vi "VNA_OPEN.vi"(8 "error in (no error)":errorcluster, 9 "Clear Error w/ Report?":bool, 10 "Configuration Cluster":T1={"General"={"Config.ini"=path "", "Default Logging Path"=path ""}, "Hardware"={"Global T VAR"="", "Global B VAR"="", "VISAS"={"GEN COM"="", "SCOPE COM"="", "VNA COM"=""}, "Connected?"={"SCOPE"=FALSE, "GEN"=FALSE, "VNA"=FALSE}}, "Operation"={"Operation Mode"=enum."Idle-Off", "Status"="", "NewLog?"=FALSE, "OvenWarn"=FALSE, "Scope Settings"={"TimeBase"=0.0, "VerticalScale"=4.0, "Channel"=enum."Channel 2"}, "Gen Settings"={"Amplitude"=0.0, "Frequency"=0.0, "Offset"=0.0}}}) -> (0 "error out":errorcluster, 1 "Success?":bool, 2 "Configuration Cluster Out":T1={"General"={"Config.ini"=path "", "Default Logging Path"=path ""}, "Hardware"={"Global T VAR"="", "Global B VAR"="", "VISAS"={"GEN COM"="", "SCOPE COM"="", "VNA COM"=""}, "Connected?"={"SCOPE"=FALSE, "GEN"=FALSE, "VNA"=FALSE}}, "Operation"={"Operation Mode"=enum."Idle-Off", "Status"="", "NewLog?"=FALSE, "OvenWarn"=FALSE, "Scope Settings"={"TimeBase"=0.0, "VerticalScale"=4.0, "Channel"=enum."Channel 2"}, "Gen Settings"={"Amplitude"=0.0, "Frequency"=0.0, "Offset"=0.0}}}, 4 "message":string)   [LabVIEW 2021]
uses:
  Config_Cluster.ctl
  Mode_Enum.ctl
  <vilib>/Utility/error.llb/DialogType.ctl
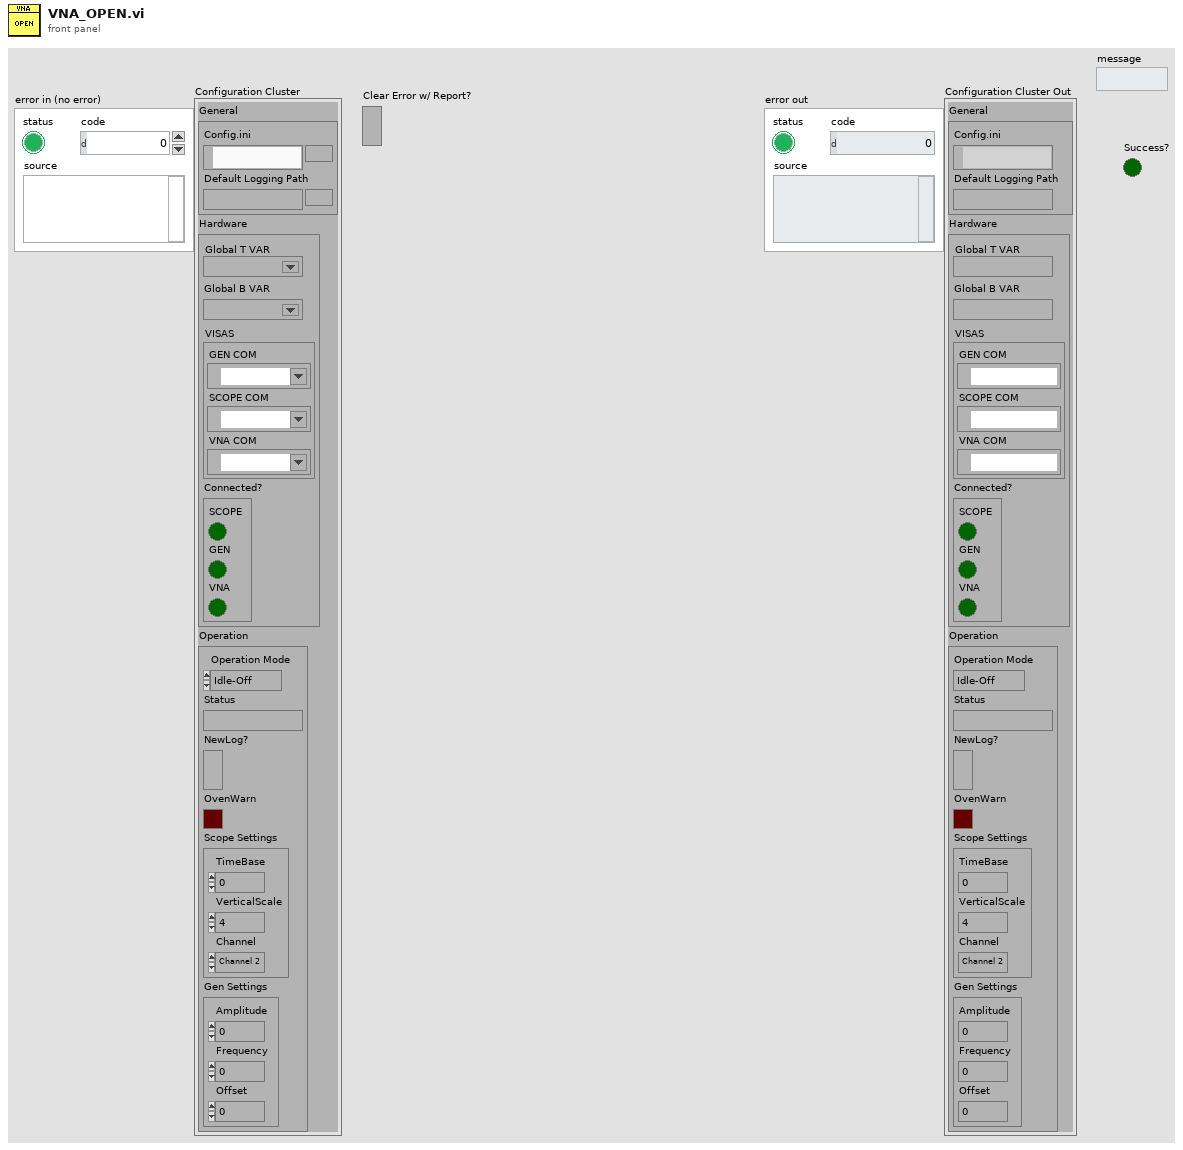
[diagram p1: front panel]
types:
  T1 = typedef "Config_Cluster.ctl" = cluster{"General":cluster{"Config.ini":path, "Default Logging Path":path}, "Hardware":cluster{"Global T VAR":refnum<k21>, "Global B VAR":refnum<k21>, "VISAS":cluster{"GEN COM":refnum<visa-resource-name>, "SCOPE COM":refnum<visa-resource-name>, "VNA COM":refnum<visa-resource-name>}, "Connected?":cluster{"SCOPE":bool, "GEN":bool, "VNA":bool}}, "Operation":cluster{"Operation Mode":T2, "Status":string, "NewLog?":bool, "OvenWarn":bool, "Scope Settings":cluster{"TimeBase":dbl, "VerticalScale":dbl, "Channel":enum16{"Channel 2", "Channel 1"}}, "Gen Settings":cluster{"Amplitude":dbl, "Frequency":dbl, "Offset":dbl}}}
  T2 = typedef "Mode_Enum.ctl" = enum16{"Logging", "Idle-Off", "Idle"}
  T3 = typedef "DialogType.ctl" = u16
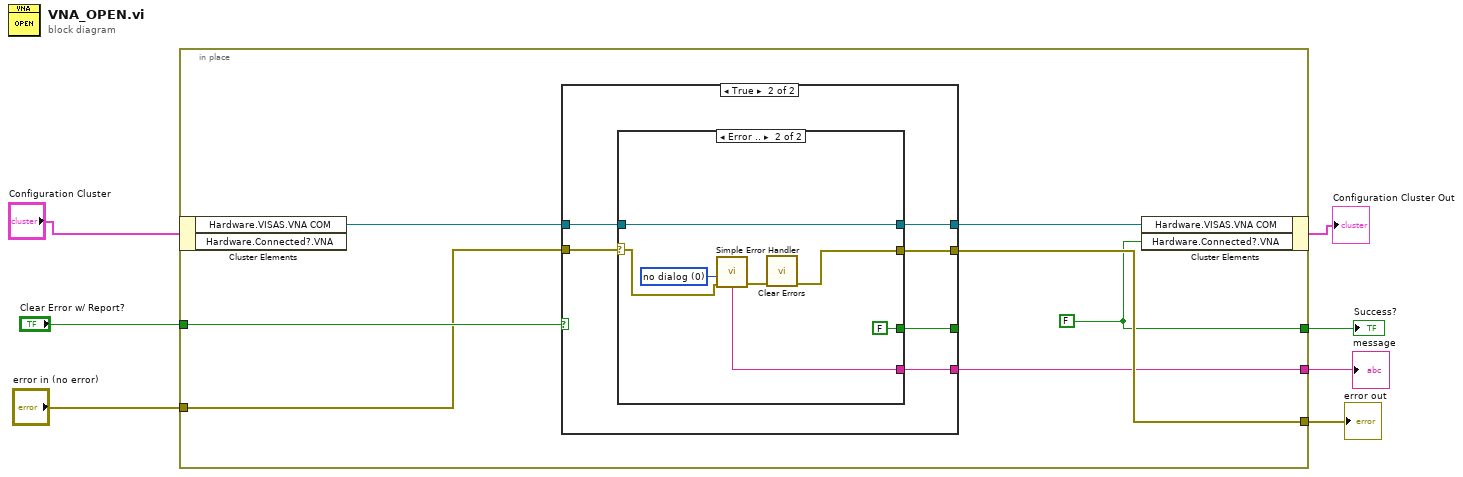
[diagram p0: block diagram]
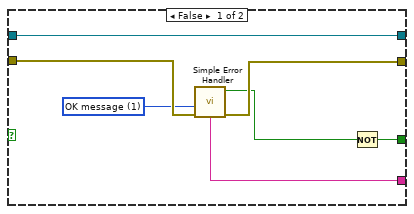
[diagram p2: hidden frame]
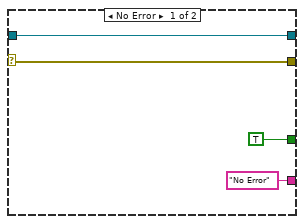
[diagram p3: hidden frame]
diagram:
  n1 = in-place {
    in-place-border: "error in (no error)" -> [w9]
    in-place-border: [w12] -> w4
    in-place-border: "Clear Error w/ Report?" -> [w14]
    in-place-border: [w8] -> w2
    in-place-border: [w11] -> w1
    w8 = FALSE
    n2 = in-place-cluster #1("Configuration Cluster") -> ("Hardware.VISAS.VNA COM"=w10:refnum<visa-resource-name>)  [unwired: 1 out]
    n3 = case shown="True" w14 {
      tunnel: w9 -> [w20 w27]
      tunnel: w10 -> [w21 w26]
      tunnel: [w18 w25] -> _
      tunnel: [w21 w24] -> w13
      tunnel: [w19 w23] -> w12
      tunnel: [w15 w22] -> w11
      frame False {
        w16 = T3 1 items=["no dialog", "OK message", "continue or stop message", "OK message + warnings", "continue/stop + warnings"] ("type of dialog (OK msg:1)")
        n4 = call <vilib>:"Simple Error Handler.vi"("type of dialog (OK msg:1)"=w16, "error in (no error)"=w20) -> ("error?"=w17:bool, "error out"=w19:errorcluster, "message"=w15:string)  [unwired: 3 in, 2 out]
        n5 = Not(x=w17) -> (.not. x?=w18:bool)
      }
      frame True {
        n6 = case shown="Error .." w27 {
          selector: w27 -> [w29 w35]
          tunnel: w26 -> [w30 w37]
          tunnel: [TRUE FALSE] -> w25
          tunnel: [w30 w37] -> w24
          tunnel: [w29 w33] -> w23
          tunnel: ["No Error" ("message") w32] -> w22
          frame No Error {
          }
          frame Error {
            w36 = T3 0 items=["no dialog", "OK message", "continue or stop message", "OK message + warnings", "continue/stop + warnings"] ("type of dialog (OK msg:1)")
            n7 = call <vilib>:"Simple Error Handler.vi"("type of dialog (OK msg:1)"=w36, "error in (no error)"=w35) -> ("error out"=w34:errorcluster, "message"=w32:string)  [unwired: 3 in, 3 out]
            n8 = call <vilib>:"Clear Errors.vi"("error in (no error)"=w34) -> ("error out"=w33:errorcluster)  [unwired: 5 in, 1 out]
          }
        }
      }
    }
    n9 = in-place-cluster #1("Hardware.VISAS.VNA COM"=w13, "Hardware.Connected?.VNA"=w8) -> (→"Configuration Cluster Out":T1)
  }
  "error out" <- w4
  "Success?" <- w2
  "message" <- w1
